vi "场景列表删除场景.vi"(8 "模式列表 new":T1(array[cluster]) {"sce-pannel-list"."pannel"."ID" format="%02x"}, 10 "场景":string, 11 "模式列表":T2(array[cluster])) -> (0 "模式列表 new output":T1(array[cluster]) {"sce-pannel-list"."pannel"."ID" format="%02x"}, 3 "模式列表-output":T2(array[cluster]))   [LabVIEW 2019]
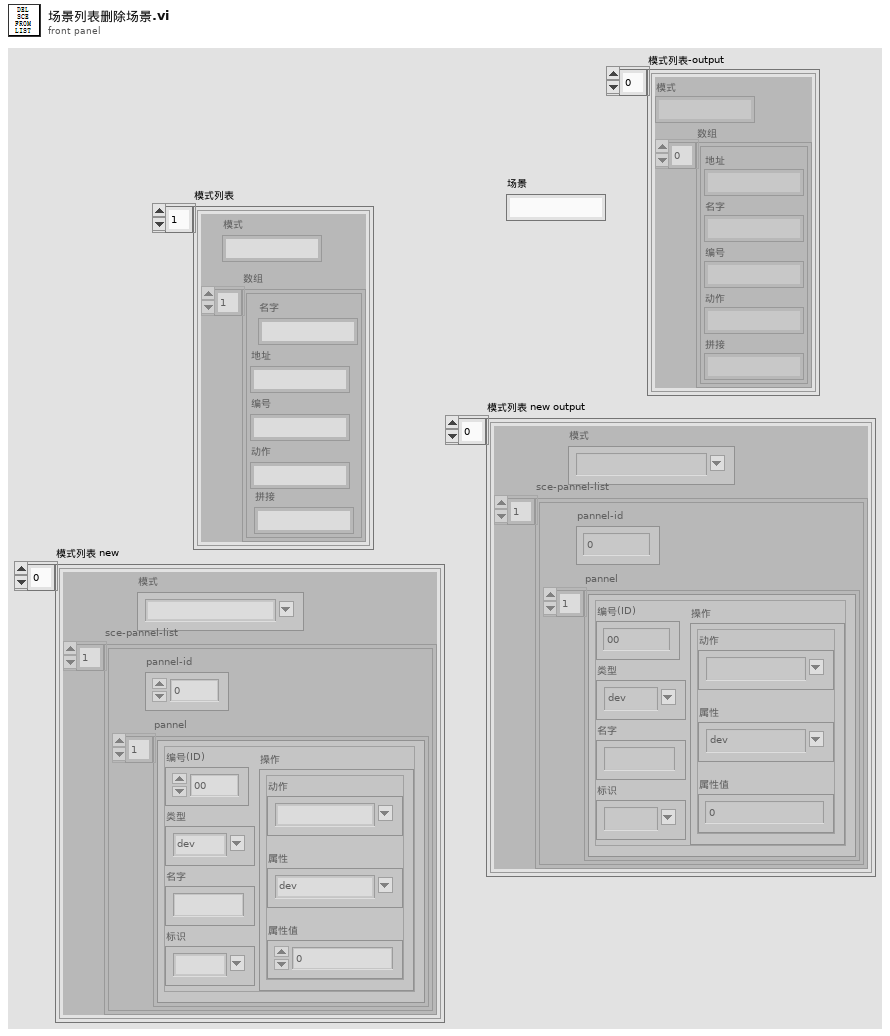
[diagram p1: front panel]
types:
  T1 = cluster{"模式":string, "sce-pannel-list":cluster{"pannel":cluster{"ID":u8, "type":string, "flag":string, "name":string, "Act":cluster{"Attribute":string, "Action":string, "Value":dbl}}[], "pannel-id":dbl}[]}[]
  T2 = cluster{"模式":string, "数组":cluster{"地址":string, "名字":string, "编号":string, "动作":string, "拼接":string}[]}[]
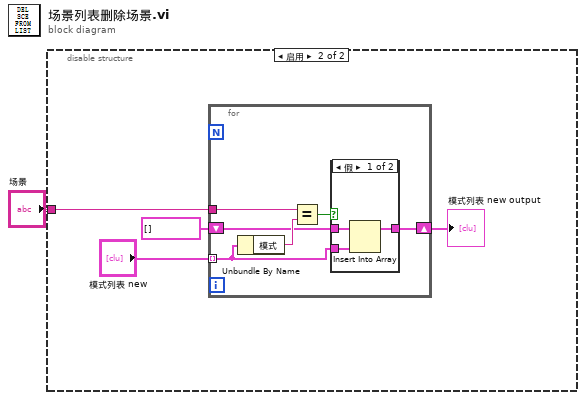
[diagram p0: block diagram]
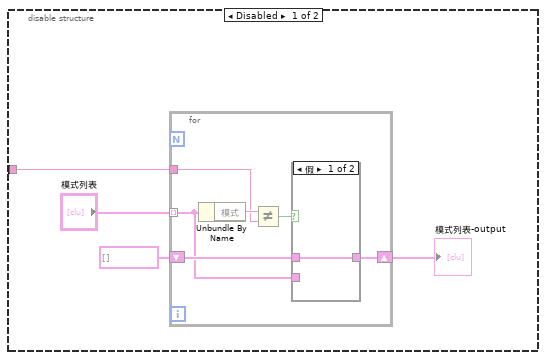
[diagram p2: hidden frame]
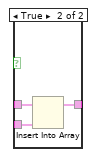
[diagram p3: hidden frame]
diagram:
  n1 = disable-structure shown="启用" {
    disable-tunnel: "场景" -> [w2 w18]
    frame Disabled {
      n2 = for {
        tunnel: "模式列表" -> [w9] mode=indexing
        shift-right: [w11] -> w3
        shift-left: T2 [] -> [w10]
        tunnel: w2 -> [w7]
        n3 = Unbundle By Name(w9) -> ("模式"=w8:string)
        n4 = Not Equal?(x=w8, y=w7) -> (x != y?=w6:bool)
        n5 = case shown="假" w6 {
          tunnel: [w12 w15] -> w11
          tunnel: w10 -> [w12 w14]
          tunnel: w9 -> [_ w13]
          frame False {
          }
          frame True {
            n6 = Insert Into Array(array=w14, new element=w13) -> (w15:T2)  [unwired: 1 in]
          }
        }
      }
      "模式列表-output" <- w3
    }
    frame Enabled {
      n7 = for {
        tunnel: "模式列表 new" -> [w23] mode=indexing
        tunnel: w18 -> [w25]
        shift-right: [w22] -> w17
        shift-left: T1 [] -> [w21]
        n8 = Unbundle By Name(w23) -> ("模式"=w24:string)
        n9 = Equal?(x=w25, y=w24) -> (x = y?=w20:bool)
        n10 = case shown="假" w20 {
          tunnel: w23 -> [w28 _]
          tunnel: [w27 w29] -> w22
          tunnel: w21 -> [w26 w29]
          frame False {
            n11 = Insert Into Array(array=w26, new element=w28) -> (w27:T1)  [unwired: 1 in]
          }
          frame True {
          }
        }
      }
      "模式列表 new output" <- w17
    }
  }
